vi "Flyback.vi"(6 "Flyback Time [Clock Cycles]":u16=10, 10 "Center (V)":dbl=1.0 format="%#_13g", 11 "Amplitude (V)":dbl=1.0 format="%#_13g") -> (3 "Waveform + Flyback":dbl[](array[numeric]))   [LabVIEW 2018]
uses:
  <vilib>/Analysis/NI_AALBase.lvlib
panel:
  out "XY Graph":cluster{i32[], "sine wave":dbl[]}(graph)
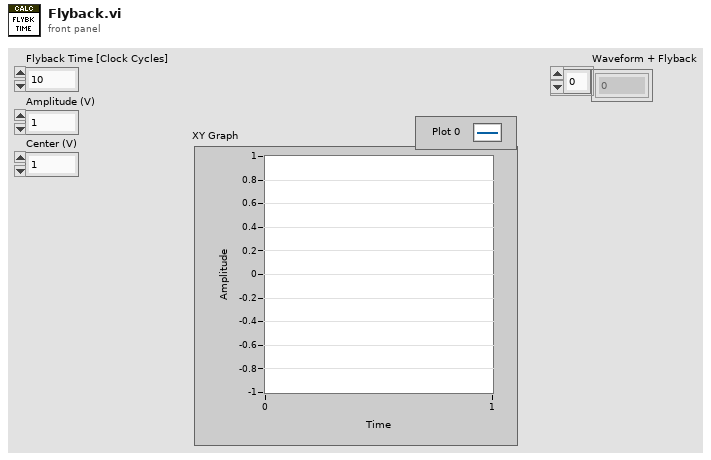
[diagram p1: front panel]
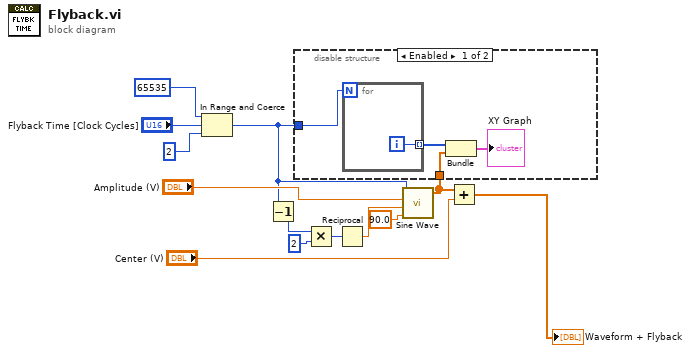
[diagram p0: block diagram]
diagram:
  n1 = In Range and Coerce(upper limit=u16 65535 ("2^x"), x="Flyback Time [Clock Cycles]", lower limit=u16 2) -> (coerced(x)=w4:u16)  [unwired: 1 out]
  n2 = Decrement(x=w4) -> (x-1=w7:u16)
  n3 = Multiply(x=w7, y=2) -> (x*y=w10:i32)
  n4 = Reciprocal(x=w10) -> (1/x=w11:dbl)
  n5 = call <vilib>:"Sine Wave.vi"("samples"=w4, "amplitude"="Amplitude (V)", "frequency"=w11, "phase in"=90.0) -> ("sine wave"=w12:dbl[])  [unwired: 1 in, 2 out]
  n6 = disable-structure shown="Enabled" {
    disable-tunnel: w12 -> [w16 _]
    disable-tunnel: w4 -> [w14 _]
    frame Enabled {
      n7 = for {
        N: w14 -> [_]
        tunnel: [w18] -> w17 mode=indexing
        i -> [w18]
      }
      n8 = Bundle(w17, "sine wave"=w16) -> (→"XY Graph":cluster{i32[], "sine wave":dbl[]})  [unwired: 1 in]
    }
    frame Disabled {
    }
  }
  n9 = Add(x=w12, y="Center (V)") -> (x+y=→"Waveform + Flyback":dbl[])
